vi "PH_Waveplate-GUI_6P.ProcEvents.vi"(0 "i ref in":refnum<vi>, 5 "error in":errorcluster) -> (14 "i ref out":refnum<vi>, 19 "error out":errorcluster)   [LabVIEW 2014, in "PH_Waveplate-GUI_6P.lvlib"]
doc: "This method is used to define the events the object will listen to. Add your own events here."
uses:
  PH_Waveplate-GUI_6P.lvlib
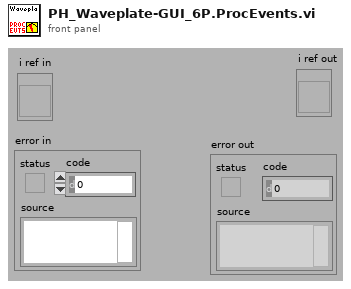
[diagram p1: front panel]
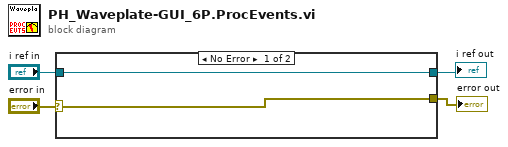
[diagram p0: block diagram]
diagram:
  n1 = case shown="No Error" "error in" {
    selector: "error in" -> [w6 w7]
    tunnel: "i ref in" -> [w5 w8]
    tunnel: [w5 w8] -> w3
    tunnel: [w6 w7] -> w2
    frame No Error {
    }
    frame Error {
    }
  }
  "i ref out" <- w3
  "error out" <- w2
